vi "Check Conditional Disables.vi"() -> ()   [LabVIEW 2019]
uses:
  <vilib>/Utility/traverseref.llb/TRef TravTarget.ctl
  <vilib>/Utility/miscctls.llb/LVMapReplaceAction.ctl
  <vilib>/Utility/traverseref.llb/VI Scripting - Traverse.lvlib
panel:
  out "Map":map{string[], set{path}}(c390)
  out "Checking/Updating...":path
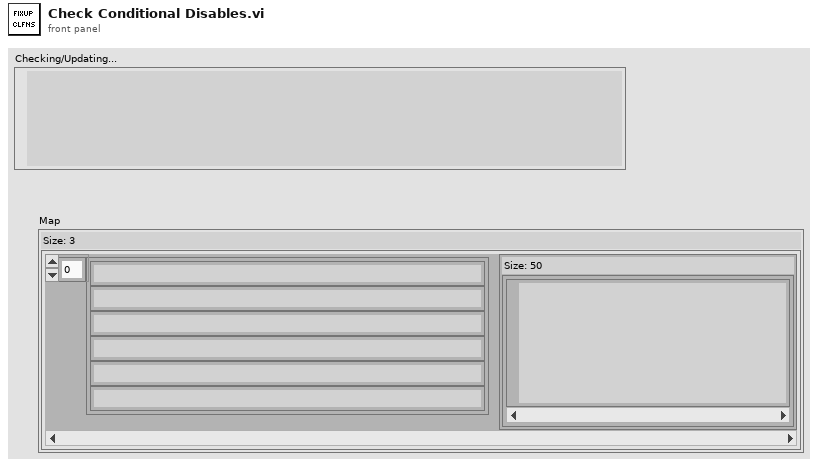
[diagram p1: front panel]
types:
  T1 = typedef "TRef TravTarget.ctl" = enum16{"FP", "BD", "Other"}
  T2 = typedef "LVMapReplaceAction.ctl" = enum32{"Modify Entry only if found", "Add or Modify Entry", "Delete Entry"}
  T3 = enum32{"Conditional Disable Style", "Diagram Disable Style", "Type Specialization Style"}
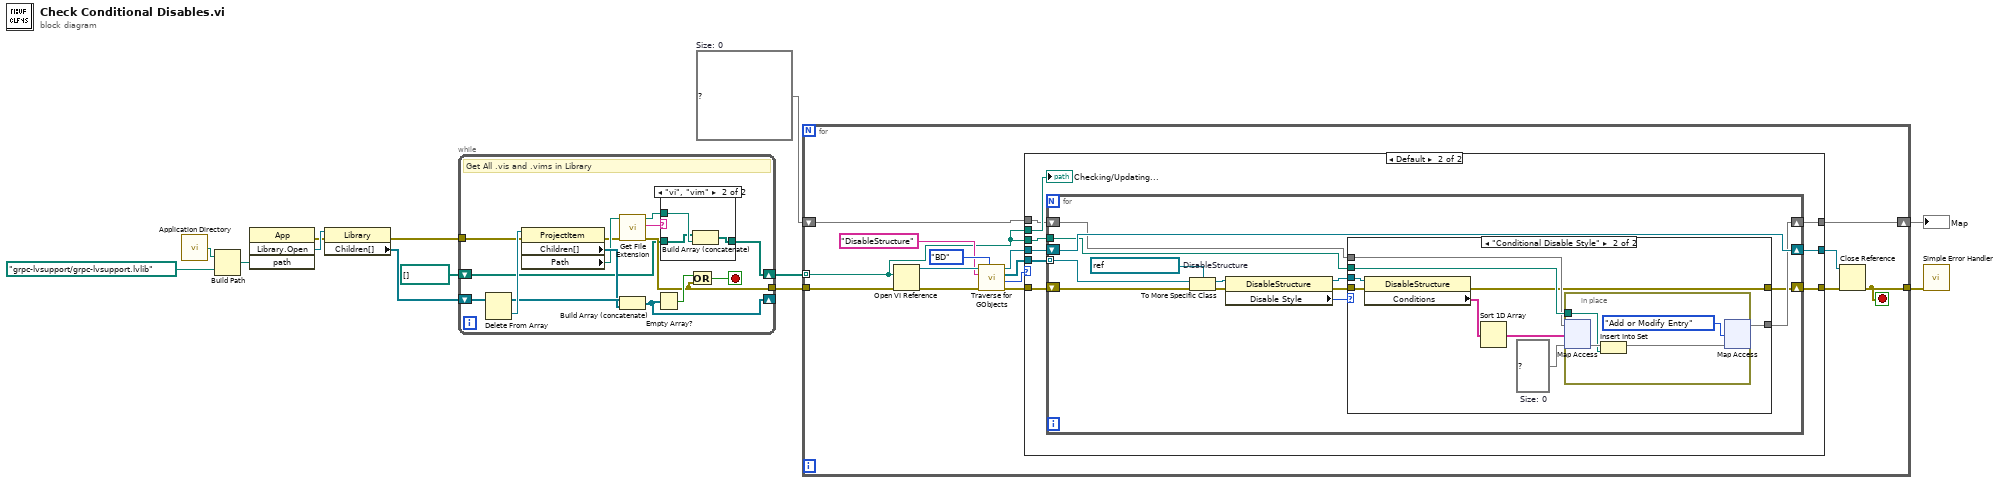
[diagram p0: block diagram]
diagram:
  w2 = map{string[], set{path}} {}  # Size: 0
  n1 = call <vilib>:"Application Directory.vi"() -> ("Application Directory"=w13:path)
  n2 = Build Path(base path=w13, name or relative path=path "grpc-lvsupport/grpc-lvsupport.lvlib") -> (appended path=w11:path)
  n3 = invoke class="App" method="Library.Open"("path"=w11) -> (error out=w8:errorcluster, "Open Library"=w10:refnum<vi>)  [unwired: 3 in, 2 out]
  n4 = property class="Library"(reference=w10, error in=w8) -> (error out=w7:errorcluster, "Children[]"=w9:refnum<vi>[])  [unwired: 1 out]
  n5 = while {
    shift-right: [w24] -> _
    shift-left: w9 -> [w28]
    tunnel: w7 -> [w19]
    tunnel: [w16] -> w4
    shift-right: [w14] -> w5
    shift-left: path[] [] ("appended array") -> [w15]
    stop <- w17 stop-if-true
    # "Get All .vis and .vims in Library"
    n6 = Delete From Array(array=w28) -> (deleted portion=w27:refnum<vi>, array with subset deleted=w26:refnum<vi>[])  [unwired: 2 in]
    n7 = property class="ProjectItem"(reference=w27, error in=w19) -> (error out=w18:errorcluster, "Children[]"=w25:refnum<vi>[], "Path"=w22:path)  [unwired: 1 out]
    n8 = call <vilib>:"Get File Extension.vi"("error in (no error)"=w18, "file"=w22) -> ("error out"=w16:errorcluster, "lowercase file extension"=w21:string, "dup file"=w20:path)  [unwired: 5 in, 2 out]
    n9 = Build Array (concatenate)(w26, w25) -> (w24:refnum<vi>[])
    n10 = Empty Array?(array=w24) -> (empty?=w23:bool)
    n11 = case shown="\"vi\", \"vim\"" w21 {
      tunnel: w20 -> [_ w32]
      tunnel: w15 -> [w29 w31]
      tunnel: [w29 w30] -> w14
      frame Default {
      }
      frame "vi", "vim" {
        n12 = Build Array (concatenate)(w31, w32) -> (w30:path[])
      }
    }
    n13 = Or(x=w23, y=w16) -> (x .or. y?=w17:bool)
  }
  n14 = for {
    tunnel: w5 -> [w35] mode=indexing
    tunnel: w4 -> [w47]
    tunnel: [w36] -> w3
    shift-right: [w34] -> w1
    shift-left: w2 -> [w33]
    stop <- w36 stop-if-true
    n15 = Open VI Reference(vi path=w35, error in (no error)=w47) -> (vi reference=w46:refnum<vi>, error out=w45:errorcluster)  [unwired: 4 in]
    n16 = call <vilib>:"Traverse for GObjects.vi"("Traverse Target"=TRef_TravTarget."BD", "error in (no error)"=w45, "Class Name"="DisableStructure", "VI Refnum"=w46) -> ("error out"=w42:errorcluster, "# of Refs"=w39:i32, "References"=w43:refnum<vi>[], "dup VI Refnum"=w40:refnum<vi>)  [unwired: 4 in]
    n17 = case shown="Default" w39 {
      tunnel: w43 -> [_ w59]
      tunnel: w42 -> [w49 w58]
      tunnel: w40 -> [w50 w57]
      tunnel: [w50 w56] -> w37
      tunnel: [w49 w55] -> w38
      tunnel: w35 -> [_ w54]
      tunnel: w35 -> [_ w53]
      tunnel: [w48 w52] -> w34
      tunnel: w33 -> [w48 w51]
      frame ..0 {
      }
      frame Default {
        n18 = for {
          tunnel: w59 -> [w72] mode=indexing
          shift-right: [w69] -> w56
          shift-left: w57 -> [w69]
          shift-right: [w62] -> w55
          shift-left: w58 -> [w71]
          tunnel: w53 -> [w66]
          shift-right: [w65] -> w52
          shift-left: w51 -> [w64]
          w70 = refnum<vi> refnum  # DisableStructure
          n19 = To More Specific Class(target class=w70, reference=w72, error in=w71) -> (specific class reference=w67:refnum<vi>, error out=w68:errorcluster)
          n20 = property class="DisableStructure"(reference=w67, error in=w68) -> (reference out=w60:refnum<vi>, error out=w61:errorcluster, "Disable Style"=w63:T3)
          n21 = case shown="\"Conditional Disable Style\"" w63 {
            tunnel: w66 -> [_ w83]
            tunnel: [w73 w82] -> w65
            tunnel: w64 -> [w73 w81]
            tunnel: [w74 w77] -> w62
            tunnel: w61 -> [w74 w78]
            tunnel: w60 -> [_ w79]
            frame Default {
            }
            frame "Conditional Disable Style" {
              w80 = set{path} {}  # Size: 0
              n22 = property class="DisableStructure"(reference=w79, error in=w78) -> (error out=w77:errorcluster, "Conditions"=w76:string[])  [unwired: 1 out]
              n23 = Sort 1D Array(array=w76) -> (sorted array=w75:string[])
              n24 = in-place {
                in-place-border: w83 -> [w86]
                n25 = in-place-map #1(w81, w75, w80) -> (w87:set{path})  [unwired: 1 out]
                n26 = Insert Into Set(10:w86, 11:w87) -> (3:w85:set{path})  [unwired: 1 out]
                n27 = in-place-map #1(w85, LVMapReplaceAction."Add or Modify Entry" ("action")) -> (w82:map{string[], set{path}})  [unwired: 2 out]
              }
            }
          }
        }
        "Checking/Updating..." <- w54
      }
    }
    n28 = Close Reference(reference=w37, error in (no error)=w38) -> (error out=w36:errorcluster)
  }
  "Map" <- w1
  n29 = call <vilib>:"Simple Error Handler.vi"("error in (no error)"=w3) -> ()  [unwired: 4 in, 5 out]
